vi "仪器参数改变发送 (子VI).vi"(8 "错误输入":errorcluster caption="错误输出") -> (0 "错误输出":errorcluster)   [LabVIEW 2016, in "数据传输系统-06.lvlib"]
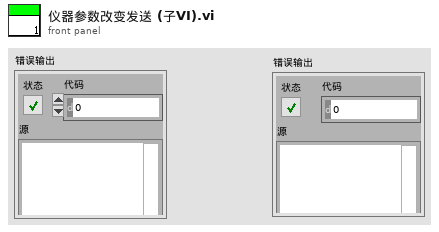
[diagram p1: front panel]
types:
  T1 = cluster{"测量量程":dbl, "测量精度":dbl, "测量间隔":dbl, "消解温度":dbl, "消解时长":dbl, "空白校准时间":timestamp, "曲线截距":dbl, "曲线斜率":dbl, "测量检出限":dbl, "测量信号值":dbl, "线性相关系数":dbl, "二次多项式系数":dbl, "标样校准时间":timestamp, "稀释倍数":dbl, "三项式系数":dbl, "空白标定系数":dbl, "量程系数":dbl, "F0/ORPA":dbl, "F1/ORPB":dbl, "F2/ORPK":dbl, "F3":dbl, "F4":dbl, "F5":dbl, "F6":dbl, "F7":dbl, "X0/滴定数":dbl, "量程":dbl}
  T2 = cluster{"CODMn关键参数":bool, "氨氮关键参数":bool, "总磷关键参数":bool, "总氮关键参数":bool, "CODCr关键参数":bool, "采配水关键参数":bool}
  T3 = cluster{"测量量程":dbl, "测量精度":dbl, "测量间隔":dbl, "消解温度":dbl, "消解时长":dbl, "空白校准时间":timestamp, "曲线截距":dbl, "曲线斜率":dbl, "测量检出限":dbl, "测量信号值":dbl, "线性相关系数":dbl, "二次多项式系数":dbl, "标样校准时间":timestamp, "稀释倍数":dbl, "三项式系数":dbl, "空白标定系数":dbl, "量程系数":dbl, "F0/ORPA":dbl, "F1/ORPB":dbl, "F2/ORPK":dbl, "F3":dbl, "F4":dbl, "F5":dbl, "F6":dbl, "F7":dbl, "X0/滴定数":dbl, "量程":dbl}[]
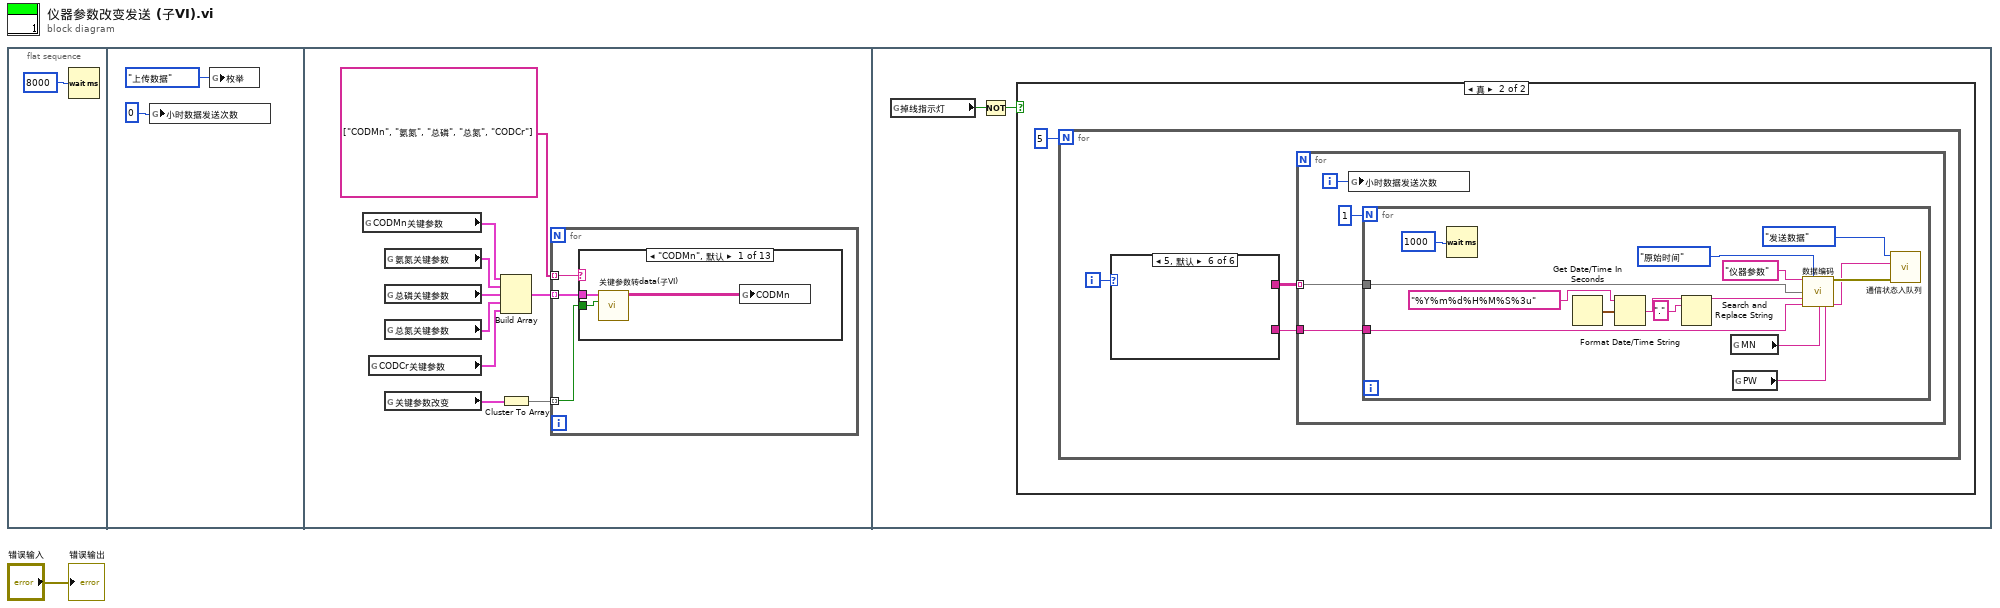
[diagram p0: block diagram]
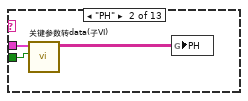
[diagram p2: hidden frame]
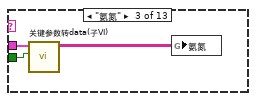
[diagram p3: hidden frame]
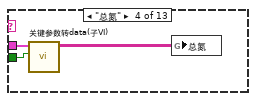
[diagram p4: hidden frame]
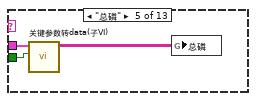
[diagram p5: hidden frame]
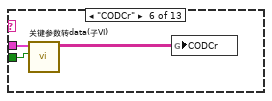
[diagram p6: hidden frame]
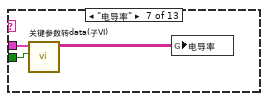
[diagram p7: hidden frame]
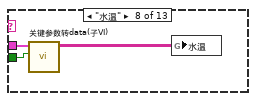
[diagram p8: hidden frame]
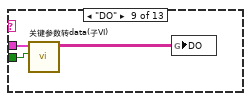
[diagram p9: hidden frame]
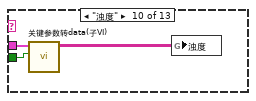
[diagram p10: hidden frame]
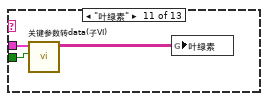
[diagram p11: hidden frame]
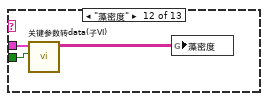
[diagram p12: hidden frame]
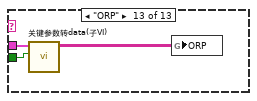
[diagram p13: hidden frame]
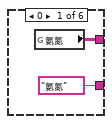
[diagram p15: hidden frame]
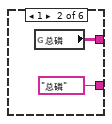
[diagram p16: hidden frame]
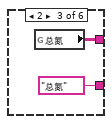
[diagram p17: hidden frame]
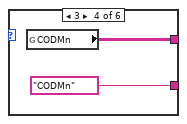
[diagram p18: hidden frame]
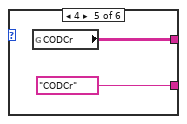
[diagram p19: hidden frame]
diagram:
  n1 = flat-sequence {
    frame #0 {
      n2 = Wait (ms)(milliseconds to wait=u32 8000 ("等待时间（毫秒）")) -> ()  [unwired: 1 out]
    }
    frame #1 {
      n3 = global write "全局 小时数据发送次数.vi" "小时数据发送次数"(0 ("小时数据发送次数")) -> ()
      n4 = global write "全局1.vi" "枚举"(enum16{"返回请求应答", "上传数据", "返回执行结果"}."上传数据" ("枚举")) -> ()
    }
    frame #2 {
      n5 = global read "全局1.vi" "CODMn关键参数"() -> (w10:T1)
      n6 = global read "全局1.vi" "CODCr关键参数"() -> (w13:T1)
      n7 = global read "全局1.vi" "氨氮关键参数"() -> (w12:T1)
      n8 = global read "全局1.vi" "总磷关键参数"() -> (w8:T1)
      n9 = global read "全局1.vi" "总氮关键参数"() -> (w7:T1)
      n10 = global read "全局1.vi" "关键参数改变"() -> (w6:T2)
      n11 = Build Array(w10, w12, w8, w7, w13) -> (w11:T3)
      n12 = Cluster To Array(cluster=w6) -> (array=w5:bool[])
      n13 = for {
        tunnel: string[] ["CODMn", "氨氮", "总磷", "总氮", "CODCr"] -> [w16] mode=indexing
        tunnel: w11 -> [w15] mode=indexing
        tunnel: w5 -> [w14] mode=indexing
        n14 = case shown="\"CODMn\", 默认" w16 {
          tunnel: w15 -> [w18 w22 w25 w28 w31 w34 w37 w40 w43 w46 w49 w52 w55]
          tunnel: w14 -> [w17 w20 w23 w26 w29 w32 w35 w38 w41 w44 w47 w50 w53]
          frame "CODMn", Default {
            n15 = call "关键参数转data(子VI).vi"("改变?"=w17, "关键参数"=w18) -> ("数组"=w19:string[][])  [unwired: 9 in]
            n16 = global write "全局 所有参数.vi" "CODMn"(w19) -> ()
          }
          frame "PH" {
            n17 = call "关键参数转data(子VI).vi"("改变?"=w20, "关键参数"=w22) -> ("数组"=w21:string[][])  [unwired: 9 in]
            n18 = global write "全局 所有参数.vi" "PH"(w21) -> ()
          }
          frame "氨氮" {
            n19 = call "关键参数转data(子VI).vi"("改变?"=w23, "关键参数"=w25) -> ("数组"=w24:string[][])  [unwired: 9 in]
            n20 = global write "全局 所有参数.vi" "氨氮"(w24) -> ()
          }
          frame "总氮" {
            n21 = call "关键参数转data(子VI).vi"("改变?"=w26, "关键参数"=w28) -> ("数组"=w27:string[][])  [unwired: 9 in]
            n22 = global write "全局 所有参数.vi" "总氮"(w27) -> ()
          }
          frame "总磷" {
            n23 = call "关键参数转data(子VI).vi"("改变?"=w29, "关键参数"=w31) -> ("数组"=w30:string[][])  [unwired: 9 in]
            n24 = global write "全局 所有参数.vi" "总磷"(w30) -> ()
          }
          frame "CODCr" {
            n25 = call "关键参数转data(子VI).vi"("改变?"=w32, "关键参数"=w34) -> ("数组"=w33:string[][])  [unwired: 9 in]
            n26 = global write "全局 所有参数.vi" "CODCr"(w33) -> ()
          }
          frame "电导率" {
            n27 = call "关键参数转data(子VI).vi"("改变?"=w35, "关键参数"=w37) -> ("数组"=w36:string[][])  [unwired: 9 in]
            n28 = global write "全局 所有参数.vi" "电导率"(w36) -> ()
          }
          frame "水温" {
            n29 = call "关键参数转data(子VI).vi"("改变?"=w38, "关键参数"=w40) -> ("数组"=w39:string[][])  [unwired: 9 in]
            n30 = global write "全局 所有参数.vi" "水温"(w39) -> ()
          }
          frame "DO" {
            n31 = call "关键参数转data(子VI).vi"("改变?"=w41, "关键参数"=w43) -> ("数组"=w42:string[][])  [unwired: 9 in]
            n32 = global write "全局 所有参数.vi" "DO"(w42) -> ()
          }
          frame "浊度" {
            n33 = call "关键参数转data(子VI).vi"("改变?"=w44, "关键参数"=w46) -> ("数组"=w45:string[][])  [unwired: 9 in]
            n34 = global write "全局 所有参数.vi" "浊度"(w45) -> ()
          }
          frame "叶绿素" {
            n35 = call "关键参数转data(子VI).vi"("改变?"=w47, "关键参数"=w49) -> ("数组"=w48:string[][])  [unwired: 9 in]
            n36 = global write "全局 所有参数.vi" "叶绿素"(w48) -> ()
          }
          frame "藻密度" {
            n37 = call "关键参数转data(子VI).vi"("改变?"=w50, "关键参数"=w52) -> ("数组"=w51:string[][])  [unwired: 9 in]
            n38 = global write "全局 所有参数.vi" "藻密度"(w51) -> ()
          }
          frame "ORP" {
            n39 = call "关键参数转data(子VI).vi"("改变?"=w53, "关键参数"=w55) -> ("数组"=w54:string[][])  [unwired: 9 in]
            n40 = global write "全局 所有参数.vi" "ORP"(w54) -> ()
          }
        }
      }
    }
    frame #3 {
      n41 = global read "全局 数据发送重叠.vi" "掉线指示灯"() -> (w57:bool)
      n42 = Not(x=w57) -> (.not. x?=w56:bool)
      n43 = case shown="真" w56 {
        frame False {
        }
        frame True {
          n44 = for {
            N: 5 -> [_]
            i -> [w61]
            n45 = case shown="5, 默认" w61 {
              tunnel: [w63 w65 w67 w69 w71 _] -> w60
              tunnel: ["氨氮" ("污染物编码") "总磷" ("污染物编码") "总氮" ("污染物编码") "CODMn" ("污染物编码") "CODCr" ("污染物编码") _] -> w59
              frame 0 {
                n46 = global read "全局 所有参数.vi" "氨氮"() -> (w63:string[][])
              }
              frame 1 {
                n47 = global read "全局 所有参数.vi" "总磷"() -> (w65:string[][])
              }
              frame 2 {
                n48 = global read "全局 所有参数.vi" "总氮"() -> (w67:string[][])
              }
              frame 3 {
                n49 = global read "全局 所有参数.vi" "CODMn"() -> (w69:string[][])
              }
              frame 4 {
                n50 = global read "全局 所有参数.vi" "CODCr"() -> (w71:string[][])
              }
              frame 5, Default {
              }
            }
            n51 = for {
              tunnel: w59 -> [w75]
              tunnel: w60 -> [w74] mode=indexing
              i -> [w73]
              n52 = global write "全局 小时数据发送次数.vi" "小时数据发送次数"(w73) -> ()
              n53 = for {
                N: 1 -> [_]
                tunnel: w75 -> [w81]
                tunnel: w74 -> [w80]
                n54 = Wait (ms)(milliseconds to wait=u32 1000 ("等待时间（毫秒）")) -> ()  [unwired: 1 out]
                n55 = Get Date/Time In Seconds() -> (seconds since 1Jan1904=w88:timestamp)
                n56 = Format Date/Time String(time format string (%c)="%Y%m%d%H%M%S%3u" ("时间格式字符串(%c)"), seconds (now)=w88) -> (date/time string=w87:string)  [unwired: 1 in]
                n57 = Search and Replace String(input string=w87, search string="." ("搜索字符串")) -> (result string=w85:string)  [unwired: 6 in, 3 out]
                n58 = global read "断电保存全局.vi" "MN"() -> (w84:string)
                n59 = global read "断电保存全局.vi" "PW"() -> (w83:string)
                n60 = call "数据编码.vi"("table输入"="仪器参数" ("新元素/子数组"), "仪器参数上传时间"=enum16{"精确到小时", "原始时间"}."原始时间", "仪器参数"=w80, "QN"=w85, "参数"=w81, "MN"=w84, "PW"=w83) -> ("错误常量"=w82:errorcluster, "通讯包字符串"=w76:string)  [unwired: 7 in]
                n61 = call "通信状态入队列.vi"("错误输入（无错误）"=w82, "发送报文"=w76, "枚举"=enum16{"打开连接", "发送数据", "读取数据", "数据处理", "关闭连接"}."发送数据") -> ()  [unwired: 8 in, 1 out]
              }
            }
          }
        }
      }
    }
  }
  "错误输出" <- "错误输入"
